vi "Set measurement mode.vi"(8 "error in (no error)":errorcluster, 10 "Measurement mode":u16(ring) items=["1"=1, "2"=2], 11 "VISA in":refnum<visa-resource-name>) -> (0 "error out":errorcluster, 3 "VISA out":refnum<visa-resource-name>)   [LabVIEW 2018, in "GP22_TDC_Arduinoed.lvlib"]
uses:
  GP22_TDC_Arduinoed.lvlib
panel:
  out "read buffer":string
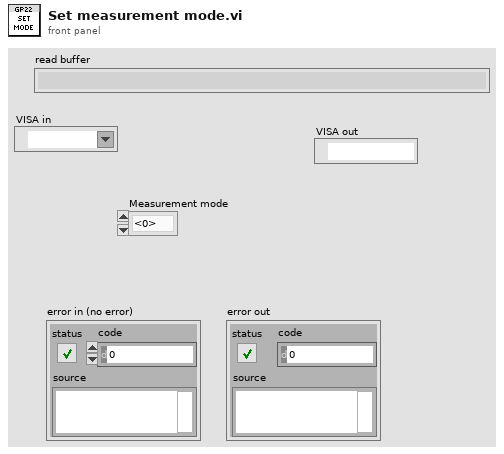
[diagram p1: front panel]
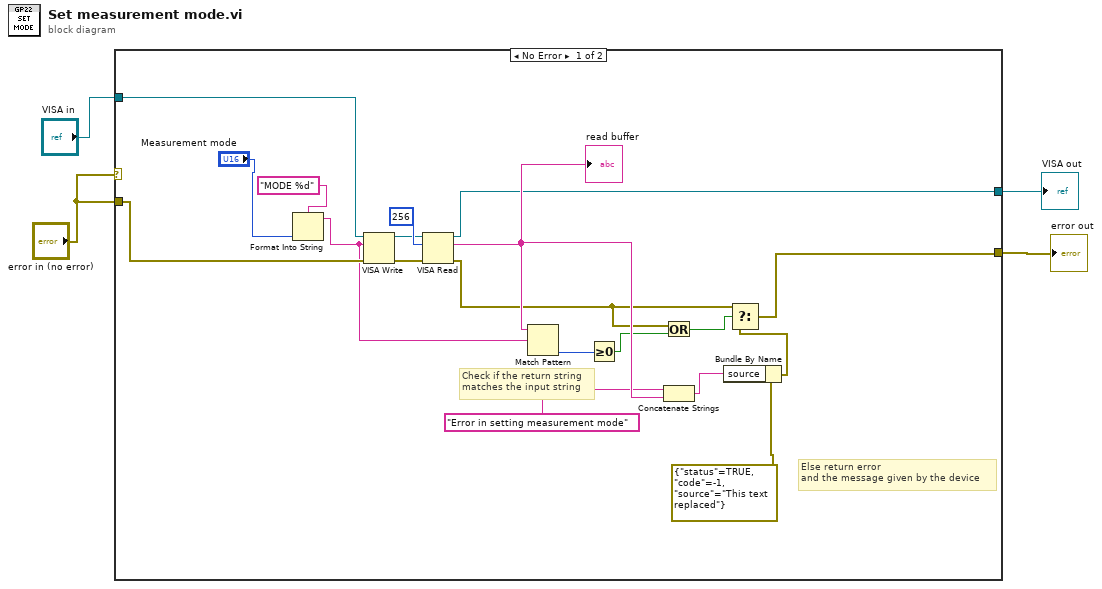
[diagram p0: block diagram]
diagram:
  n1 = case shown="No Error" "error in (no error)" {
    tunnel: [w21 w25] -> w4
    tunnel: "error in (no error)" -> [w8 w25]
    tunnel: [w10 w24] -> w2
    tunnel: "VISA in" -> [w9 w24]
    frame No Error {
      # "Else return error\nand the message given by the device"
      # "Check if the return string\nmatches the input string"
      n2 = Format Into String(format string="MODE %d" ("write buffer"), "Measurement mode") -> (resulting string=w5:string)  [unwired: 2 in, 1 out]
      n3 = VISA Write(VISA resource name=w9, write buffer=w5, error in (no error)=w8) -> (VISA resource name out=w17:refnum<visa-resource-name>, error out=w18:errorcluster)  [unwired: 1 out]
      n4 = VISA Read(VISA resource name=w17, byte count=u32 256, error in (no error)=w18) -> (VISA resource name out=w10:refnum<visa-resource-name>, read buffer=w16:string, error out=w12:errorcluster)  [unwired: 1 out]
      "read buffer" <- w16
      n5 = Match Pattern(string=w16, regular expression=w5) -> (offset past match=w20:i32)  [unwired: 1 in, 3 out]
      n6 = Greater Or Equal To 0?(x=w20) -> (x >= 0?=w13:bool)
      n7 = Or(x=w12, y=w13) -> (x .or. y?=w11:bool)
      n8 = Concatenate Strings("Error in setting measurement mode" ("string"), w16) -> (w15:string)
      n9 = Bundle By Name(cluster=errorcluster {"status"=TRUE, "code"=-1, "source"="This text replaced"} ("f"), "source"=w15) -> (w23:errorcluster)
      n10 = Select(t=w12, s=w11, f=w23) -> (s? t:f=w21:errorcluster)
    }
    frame Error {
    }
  }
  "error out" <- w4
  "VISA out" <- w2
